vi "exercise6.vi"() -> ()   [LabVIEW 2025]
panel:
  out "String 2":string
  out "String":string
  in  "Numeric":dbl
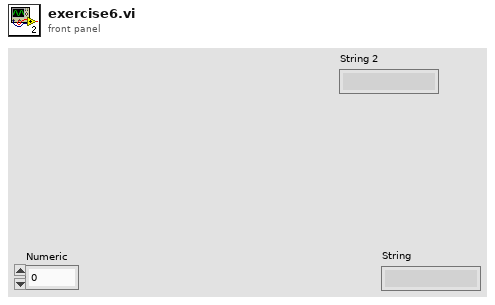
[diagram p1: front panel]
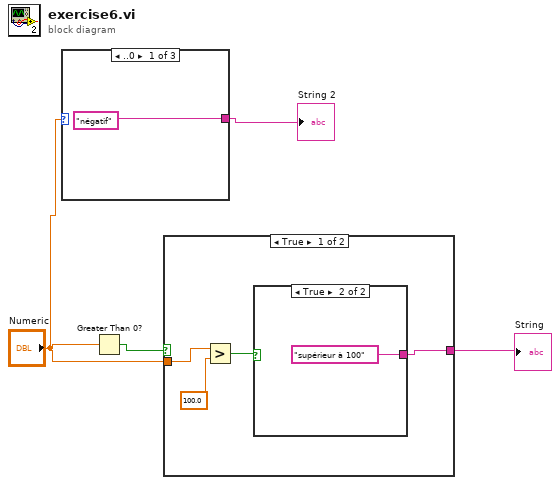
[diagram p0: block diagram]
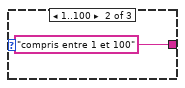
[diagram p2: hidden frame]
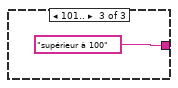
[diagram p3: hidden frame]
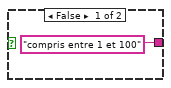
[diagram p4: hidden frame]
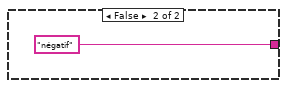
[diagram p5: hidden frame]
diagram:
  n1 = case shown="..0" "Numeric" {
    tunnel: ["négatif" "compris entre 1 et 100" "supérieur à 100"] -> w1
    frame ..0 {
    }
    frame 1..100 {
    }
    frame 101.. {
    }
  }
  "String 2" <- w1
  n2 = Greater Than 0?(x="Numeric") -> (x > 0?=w4:bool)
  n3 = case shown="True" w4 {
    tunnel: "Numeric" -> [w9 _]
    tunnel: [w8 "négatif"] -> w3
    frame True {
      n4 = Greater?(x=w9, y=100.0) -> (0:w11:bool)
      n5 = case shown="True" w11 {
        tunnel: ["compris entre 1 et 100" "supérieur à 100"] -> w8
        frame False {
        }
        frame True {
        }
      }
    }
    frame False {
    }
  }
  "String" <- w3
